vi "MAIN_call.vi"(8 "error IO":errorcluster, 9 "Coordenadas_estacion_input":T1, 10 "Modo":T2=enum."MOVIMIENTO MANUAL", 11 "VISA SESSION":refnum<visa-resource-name>) -> (0 "error out":errorcluster, 2 "Coordenadas_estacion_outpu":T1)   [LabVIEW 2019]
uses:
  Typedefs/Distancia_Z.ctl
  Typedefs/Tipo_movimiento.ctl
  Typedefs/ESTADOS.ctl
  LABVIEW_ROBOT_MASTER/Type_defs/TAREAS_ROBOT.ctl
  LVPROJ_CONFIG_ESTACION/Type_defs/Coordenadas_estacion.ctl
  Typedefs/Distancia.ctl
  Typedefs/Cluster_tracking.ctl
  Typedefs/Cluster_refs_controles.ctl
  SHARED TYPES/Acciones_UI.ctl
  LVPROJ_CONFIG_ESTACION/Type_defs/coordenada_elegida.ctl
  Typedefs/Comandos.ctl
  Typedefs/Estados_arduino.ctl
  <vilib>/Utility/error.llb/Error Cluster From Error Code.vi
  <vilib>/ErrorRing/Error Ring.xnode
  SHARED TYPES/SHARED TYPES.lvlib
  SHARED VI'S/SHARED VI'S.lvlib
panel:
  in  "TabDepuracion":enum32{"Page 1", "Page 2"}(tab)
  out "Config estación?":bool
  in  "Tab Control":enum32{"Page 1"}(tab)
  in  "Set coord. NOK":bool
  in  "Set coord. OK":bool
  in  "Set coord. entrada":bool
  out "Coord.Adquirida Z":u32
  out "Coord.Adquirida Y":u32
  out "Coord.Adquirida X":u32
  in  "Set coord. socket":bool
  out "Tracking_Z":u32
  in  "Distancia Z":T3=32000 items=["2cm"=64000, "1cm"=32000, "1mm"=3200, "0.5mm"=1600, "0.2mm"=640, "0.1mm"=320, "0.05mm"=160]
  out "Movimiento ejecutado?":bool caption="MOVIMIENTO NO EJECUTADO"
  out "Tracking_Y":u32
  out "Tracking_X":u32
  out "TRAMA DE MOVIMIENTO ENVIADA":string
  out "MENSAJES AL USUARIO":string
  in  "COMENZAR MOVIMIENTO":bool
  in  "HOME":bool
  in  "Avance":bool
  in  "Retroceso":bool
  in  "Derecha":bool
  in  "Izquierda":bool
  in  "STOP PROGRAM":bool
  in  "Sube Z":bool
  in  "Baja Z":bool
  out "ESTADO FSM":T4
  out "MOVIMIENTO SOLICITADO":T5=enum."AVANZAR"
  in  "Distancia":T6=9100 items=["60cm"=54600, "50cm"=45500, "45cm"=40950, "40cm"=36400, "35cm"=31850, "30cm"=27300, "25cm"=22750, "20cm"=18200, "15cm"=13650, "10cm"=9100, "5cm"=4550, "2cm"=1820, "1cm"=910, "5mm"=455, "2mm"=182, "1mm"=91, "0.5mm"=45, "0.1mm"=9, "1 paso "=1]
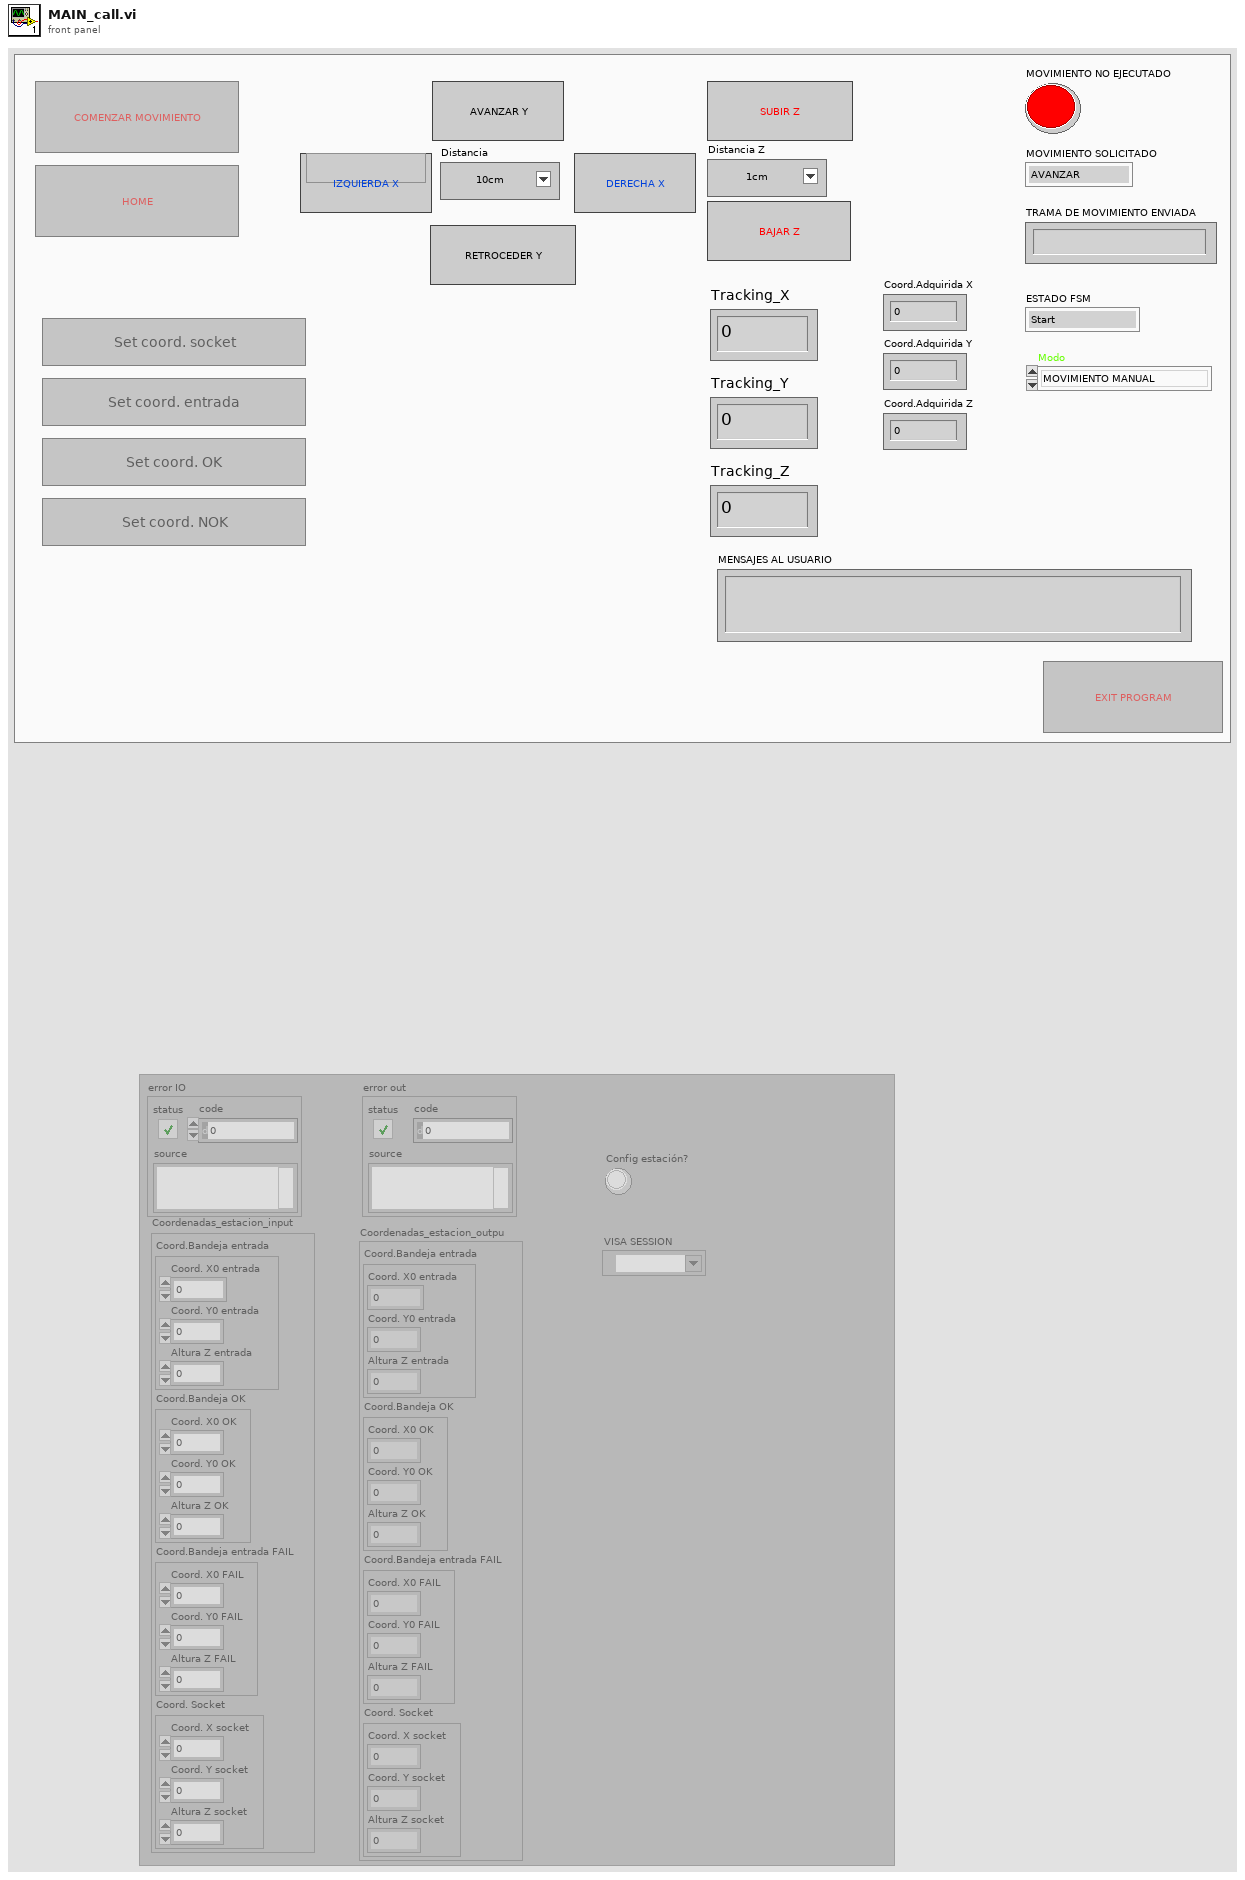
[diagram p1: front panel]
types:
  T1 = typedef "Coordenadas_estacion.ctl" = cluster{"Coord.Bandeja entrada":cluster{"Coord. X0 entrada":u32, "Coord. Y0 entrada ":u32, "Altura Z entrada":u32}, "Coord.Bandeja OK":cluster{"Coord. X0 OK":u32, "Coord. Y0 OK":u32, "Altura Z OK":u32}, "Coord.Bandeja entrada FAIL":cluster{"Coord. X0 FAIL":u32, "Coord. Y0 FAIL":u32, "Altura Z FAIL":u32}, "Coord. Socket":cluster{"Coord. X socket":u32, "Coord. Y socket":u32, "Altura Z socket":u32}}
  T2 = typedef "TAREAS_ROBOT.ctl" = enum16{"NINGUNA", "TEST ASICS", "AJUSTE CAM", "MOVER ASICS", "MOVIMIENTO MANUAL", "LEER QR", "CONFIG ESTACION"}
  T3 = typedef "Distancia_Z.ctl" = i32
  T4 = typedef "ESTADOS.ctl" = enum16{"Start", "Ping_Arduino", "Init Refs", "Check Button", "Check Limits", "Home", "Cabezal Posicion Inicio", "Terminaste posicion inicio?", "Terminar", "Salir Arduino", "Envio Parametros Movimiento", "Recepcion Comando?", "Terminaste Movimiento?", "Adquirir Coordenada", "Terminaste Home?", "Salir"}
  T5 = typedef "Tipo_movimiento.ctl" = enum16{"NINGUNO", "AVANZAR", "RETROCEDER", "DERECHA", "IZQUIERDA", "SUBIRZ", "BAJARZ", "HOME", "HOME_Z"}
  T6 = typedef "Distancia.ctl" = i32
  T7 = typedef "SHARED TYPES.lvlib/Acciones_UI.ctl" = enum16{"Activar", "Desactivar", "Reiniciar default"}
  T8 = typedef "coordenada_elegida.ctl" = enum16{"Ninguna", "Coord.bandeja entrada", "Coord.bandeja OK", "Coord.bandeja FAIL", "Coord.Socket"}
  T9 = enum8{"Enabled", "Disabled", "Disabled and Grayed Out"}
  T10 = typedef "Estados_arduino.ctl" = enum16{"2", "3", "4", "5", "6", "7", "9", "8"}
  T11 = typedef "Comandos.ctl" = enum16{"H", "FH", "FM", "FI", "FX", "FY", "FZ", "I", "OK"}
  T12 = typedef "Cluster_refs_controles.ctl" = cluster{"Comenzar mov":refnum<vi>, "Home":refnum<vi>, "Izq":refnum<vi>, "Der":refnum<vi>, "Stop Program":refnum<vi>, "Avanzar":refnum<vi>, "Bajar Z":refnum<vi>, "Distancia":refnum<vi>, "Subir Z":refnum<vi>, "Retroc":refnum<vi>, "MENSAJES AL USUARIO":refnum<vi>, "Trama enviada":refnum<vi>, "Movimiento ejecutado?":refnum<vi>}
  T13 = typedef "Cluster_tracking.ctl" = cluster{"PasosAcumulados_Y":i32, "PasosAcumulados_X":i32, "PasosAcumulados_Z":i32, "Coord.Adquirida_X":i32, "Coord.Adquirida_Y":i32, "Coord.Adquirida_Z":i32}
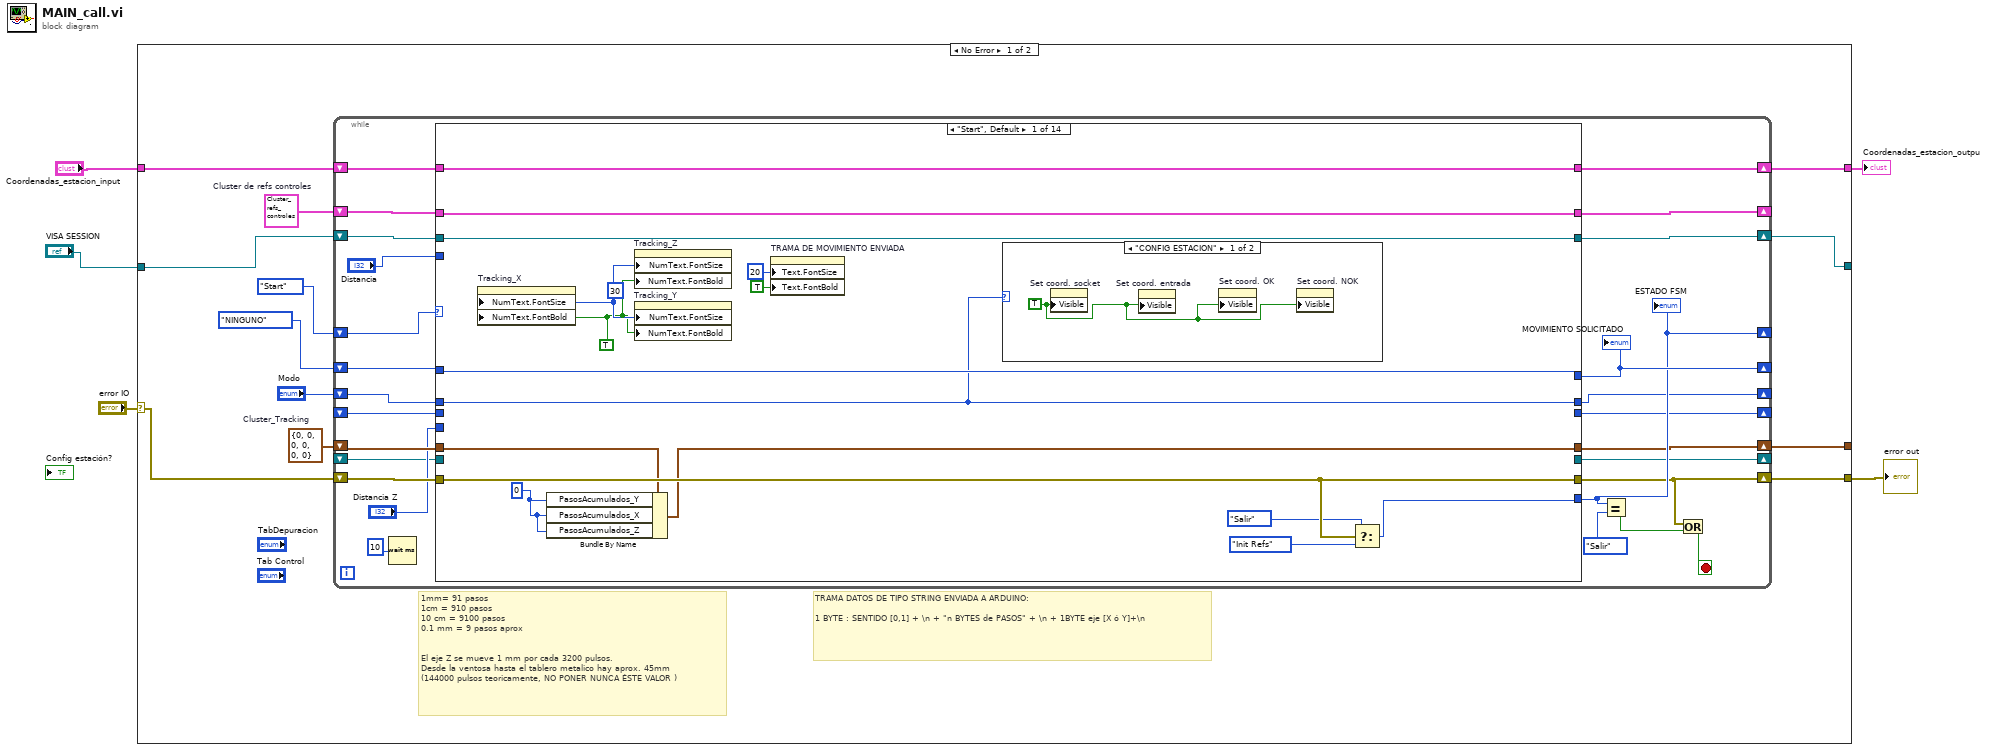
[diagram p0: block diagram]
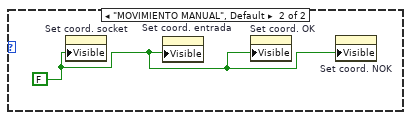
[diagram p2: hidden frame]
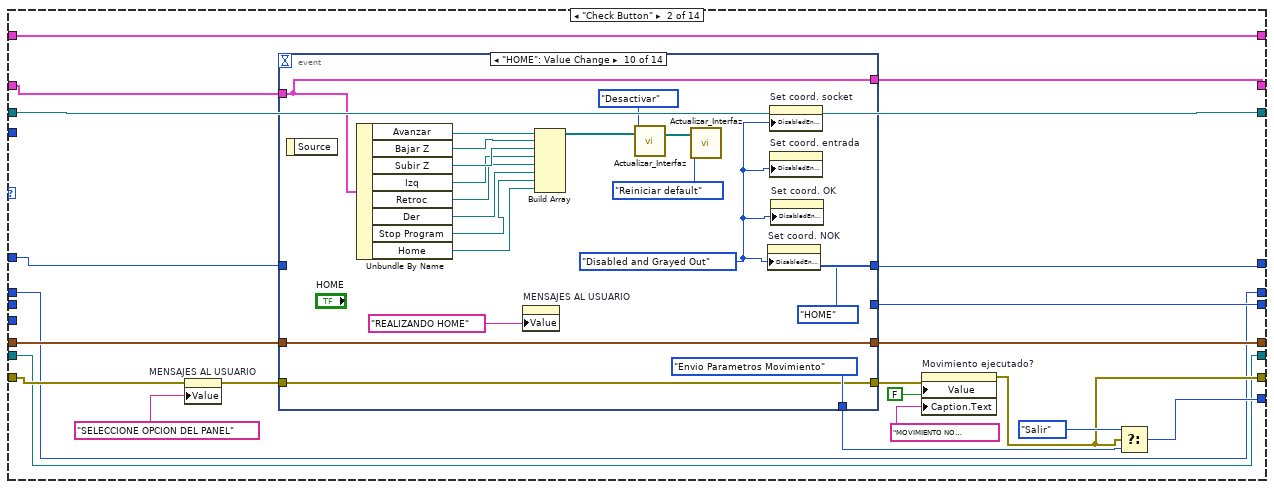
[diagram p3: hidden frame]
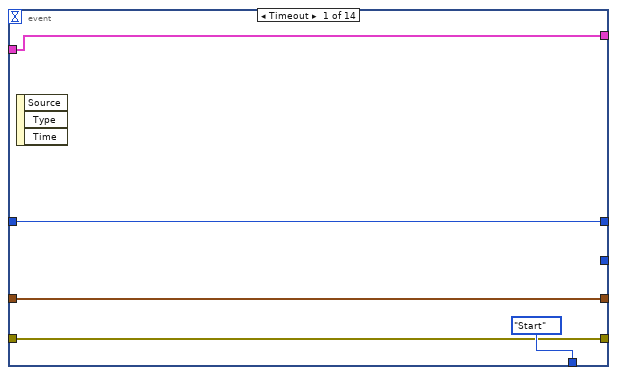
[diagram p4: hidden frame]
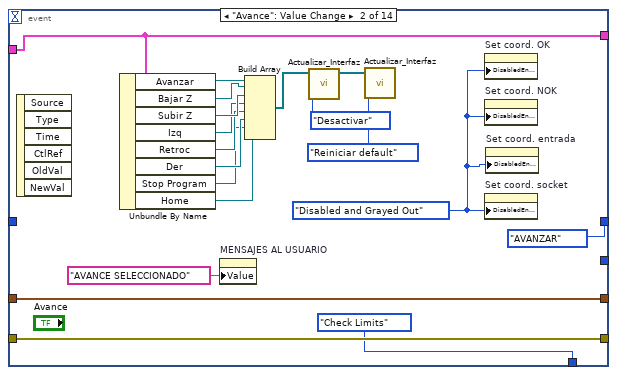
[diagram p5: hidden frame]
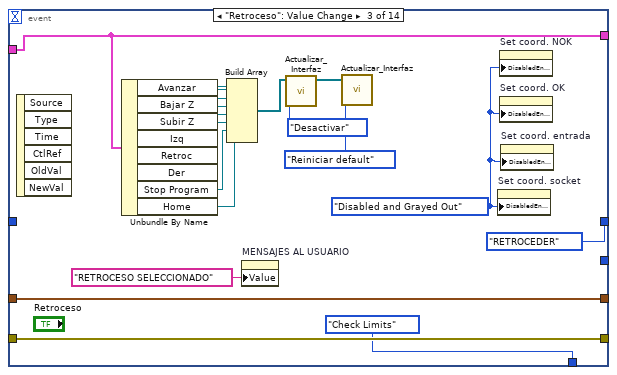
[diagram p6: hidden frame]
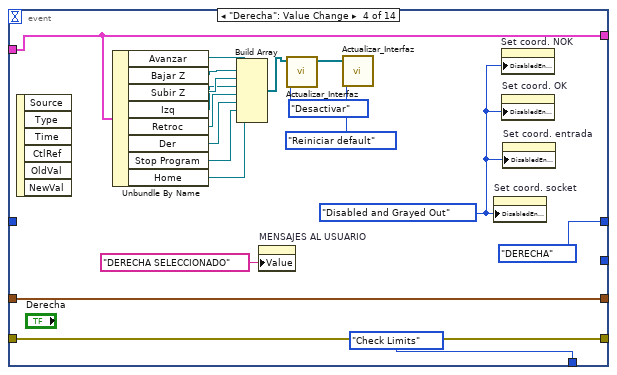
[diagram p7: hidden frame]
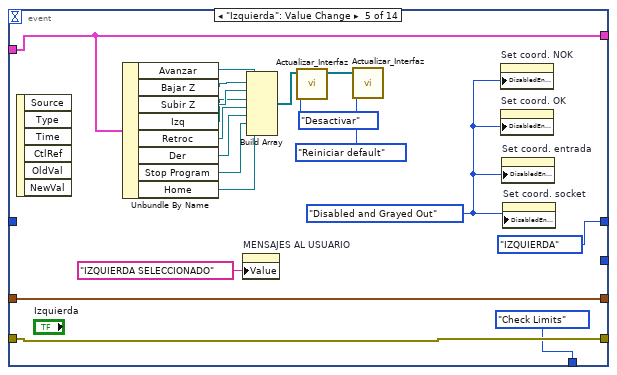
[diagram p8: hidden frame]
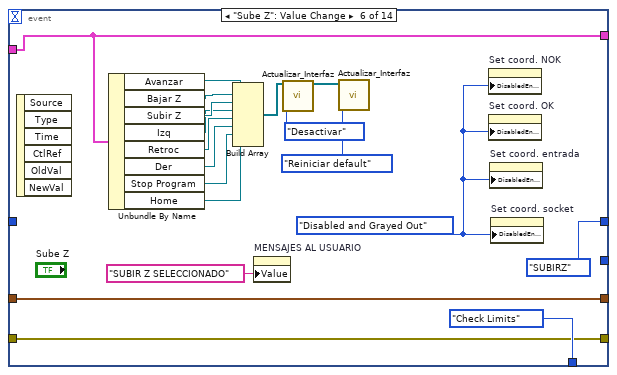
[diagram p9: hidden frame]
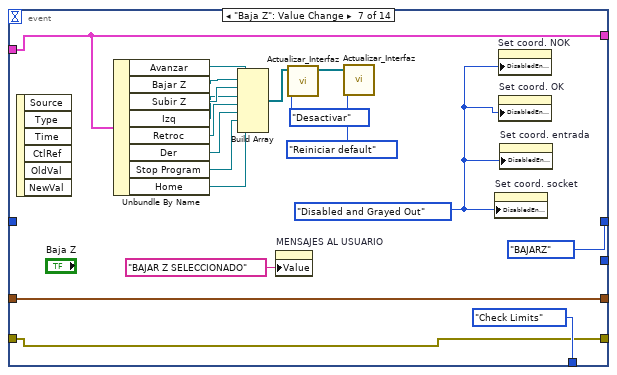
[diagram p10: hidden frame]
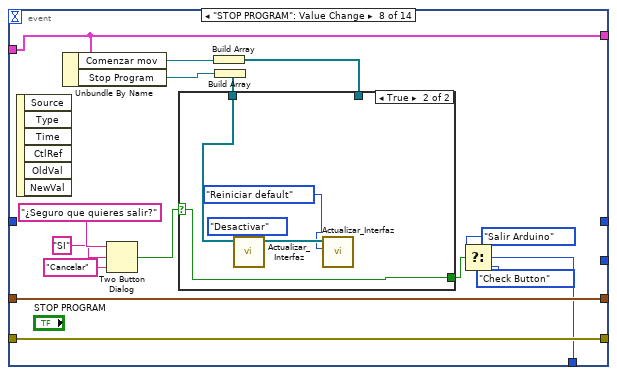
[diagram p11: hidden frame]
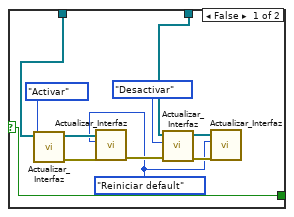
[diagram p12: hidden frame]
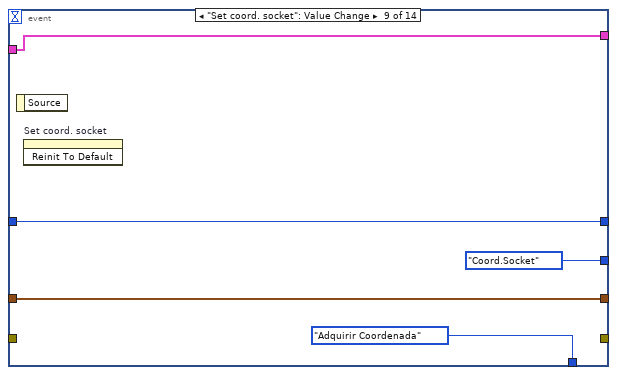
[diagram p13: hidden frame]
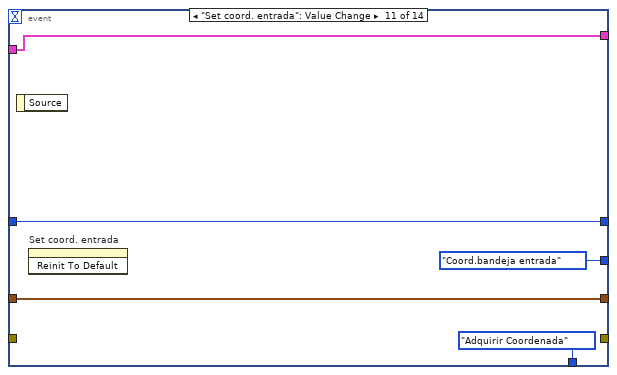
[diagram p14: hidden frame]
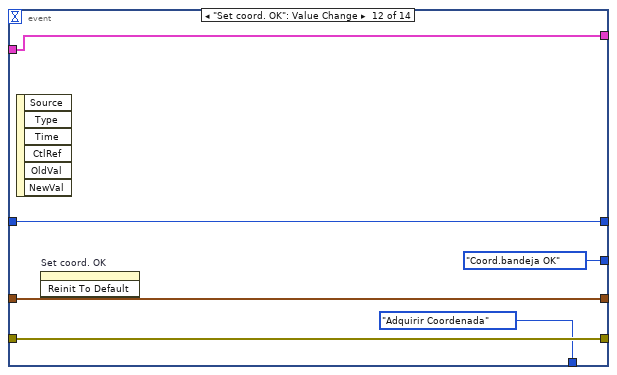
[diagram p15: hidden frame]
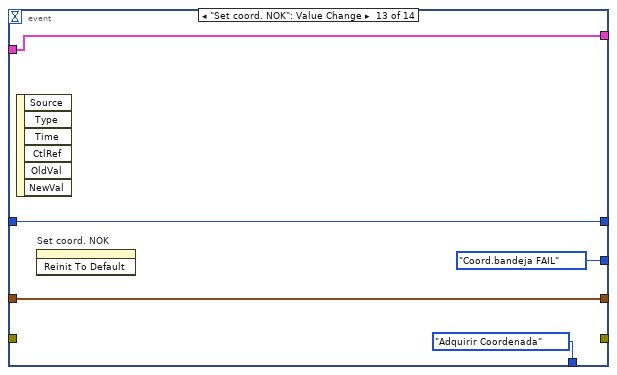
[diagram p16: hidden frame]
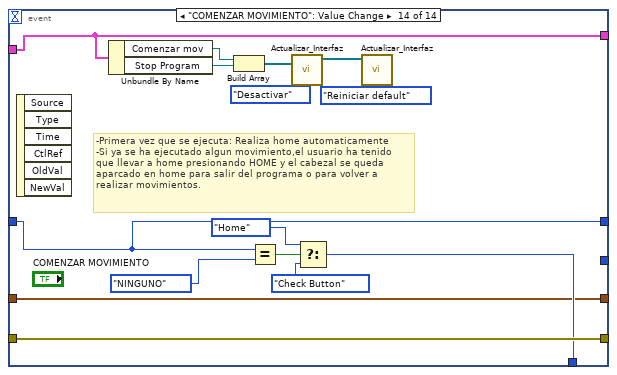
[diagram p17: hidden frame]
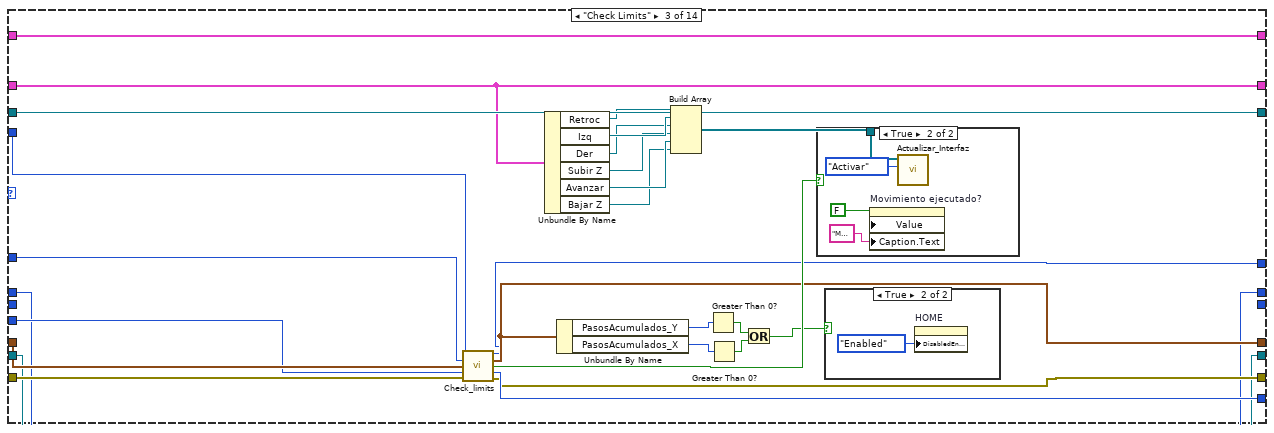
[diagram p18: hidden frame]
diagram:
  n1 = case shown="No Error" "error IO" {
    selector: "error IO" -> [w13 w731]
    tunnel: [w12 w731] -> w4
    tunnel: [w11 _] -> _
    tunnel: "Coordenadas_estacion_input" -> [w9 w730]
    tunnel: [w8 w730] -> w2
    tunnel: "VISA SESSION" -> [w7 w729]
    tunnel: [w6 w729] -> _
    frame No Error {
      w15 = T12 {"Comenzar mov"=refnum, "Home"=refnum, "Izq"=refnum, "Der"=refnum, "Stop Program"=refnum, "Avanzar"=refnum, "Bajar Z"=refnum, "Distancia"=refnum, "Subir Z"=refnum, "Retroc"=refnum, "MENSAJES AL USUARIO"=refnum, "Trama enviada"=refnum, "Movimiento ejecutado?"=refnum}  # Cluster de refs controles
      w14 = T13 {"PasosAcumulados_Y"=0, "PasosAcumulados_X"=0, "PasosAcumulados_Z"=0, "Coord.Adquirida_X"=0, "Coord.Adquirida_Y"=0, "Coord.Adquirida_Z"=0}  # Cluster_Tracking
      # "1mm= 91 pasos\n1cm = 910 pasos\n10 cm = 9100 pasos\n0.1 mm = 9 pasos aprox\n\n\nEl eje Z se mueve 1 mm por cada 3200 pulsos. \nDesde la ventosa hasta el tablero metalico hay aprox. 45mm \n(144000 pulsos teoricamente, NO PONER NUNCA ÉSTE VALOR )"
      # "TRAMA DATOS DE TIPO STRING ENVIADA A ARDUINO:\n\n1 BYTE : SENTIDO [0,1] + \\n + \"n BYTES de PASOS\" + \\n + 1BYTE eje [X ó Y]+\\n"
      n2 = while {
        shift-right: [w31] -> w12
        shift-left: w13 -> [w40]
        shift-right: [w39] -> w6
        shift-left: w7 -> [w41]
        shift-right: [w35] -> _
        shift-left: w15 -> [w36]
        shift-right: [w33] -> _
        shift-left: ESTADOS."Start" ("Enum") -> [w42]
        shift-right: [w37] -> _
        shift-left: Tipo_movimiento."NINGUNO" ("Enum") -> [w38]
        shift-right: [w28] -> w11
        shift-left: w14 -> [w29]
        shift-right: [w24] -> w8
        shift-left: w9 -> [w25]
        shift-right: [w23] -> _
        shift-left: _ -> [w22]
        shift-right: [w20] -> _
        shift-left: "Modo" -> [w26]
        shift-right: [w19] -> _
        shift-left: _ -> [w18]
        stop <- w34 stop-if-true
        n3 = Wait (ms)(milliseconds to wait=u32 10) -> ()  [unwired: 1 out]
        n4 = case shown="\"Start\", Default" w42 {
          tunnel: w41 -> [w55 w67 w314 w324 w364 w406 w449 w488 w517 w573 w593 w613 w658 w707]
          tunnel: w40 -> [w59 w66 w312 w323 w373 w405 w448 w486 w516 w569 w595 w614 w667 w706]
          tunnel: [w59 w68 w293 w331 w341 w392 w432 w486 w513 w569 w591 w612 w655 w710] -> w31
          tunnel: [w56 w79 w311 w335 w370 w402 w445 w483 w536 w570 w594 w616 w661 ESTADOS."Salir" ("f")] -> w33
          tunnel: [w55 w67 w314 w324 w364 w406 w450 w488 w537 w573 w593 w613 w658 w707] -> w39
          tunnel: w38 -> [w54 w76 w310 w336 w375 w409 w451 w487 _ _ _ _ _ w718]
          tunnel: "Distancia" -> [_ _ w313 _ _ w408 _ _ _ _ _ _ _ _]
          tunnel: [w54 w78 w291 w336 w375 w391 w444 w487 _ _ _ _ _ w718] -> w37
          tunnel: w36 -> [w50 w82 w309 w332 w361 w396 w428 w489 w531 w587 w592 w615 w660 w719]
          tunnel: [w50 w81 w309 w332 w361 w396 w428 w489 w531 w574 w592 w615 w660 w719] -> w35
          tunnel: w29 -> [w53 w75 w300 w327 w355 w389 w441 w479 w532 w564 w590 w611 w659 w717]
          tunnel: [w52 w74 w295 w327 w352 w389 w440 w478 w532 w564 w590 w611 w659 w717] -> w28
          tunnel: "Distancia Z" -> [_ _ w292 _ _ w390 _ _ _ _ _ _ _ _]
          tunnel: w26 -> [w44 w62 w288 w320 w338 w386 w410 w470 w511 w556 w588 w609 w653 w699]
          tunnel: w25 -> [w45 w65 w290 w322 w340 w388 w417 w477 w515 w559 w589 w610 w657 w704]
          tunnel: [w45 w65 w290 w322 w340 w388 w417 w473 w515 w559 w589 w610 w657 w704] -> w24
          tunnel: [_ w64 _ _ _ _ _ w472 _ _ _ _ _ _] -> w23
          tunnel: w22 -> [_ _ _ _ _ _ _ w472 _ _ _ _ _ _]
          tunnel: [w44 w62 w288 w320 w338 w386 w410 w470 w511 w556 w588 w609 w653 w699] -> w20
          tunnel: [_ w63 w289 w321 w339 w387 w411 w471 w512 _ _ _ w654 _] -> w19
          tunnel: w18 -> [_ w63 w289 w321 w339 w387 w411 w471 w512 _ _ _ _ w703]
          frame "Start", Default {
            w49 = u32 30 ("Text.Font:Size")
            w48 = TRUE ("Text.Font:Bold")
            w51 = 0 ("PasosAcumulados_Y")
            n5 = property on="Tracking_X" class="DigNum (strict)"("NumText.FontSize"=w49, "NumText.FontBold"=w48) -> ()  [unwired: 2 in, 2 out]
            n6 = Bundle By Name(cluster=w53, "PasosAcumulados_Y"=w51, "PasosAcumulados_X"=w51, "PasosAcumulados_Z"=w51) -> (w52:T13)
            n7 = property on="Tracking_Z" class="DigNum (strict)"("NumText.FontSize"=w49, "NumText.FontBold"=w48) -> ()  [unwired: 2 in, 2 out]
            n8 = property on="Tracking_Y" class="DigNum (strict)"("NumText.FontSize"=w49, "NumText.FontBold"=w48) -> ()  [unwired: 2 in, 2 out]
            n9 = property on="TRAMA DE MOVIMIENTO ENVIADA" class="Str"("Text.FontSize"=u32 20 ("Text.Font:Size"), "Text.FontBold"=TRUE ("Text.Font:Bold")) -> ()  [unwired: 2 in, 2 out]
            n10 = case shown="\"CONFIG ESTACION\"" w44 {
              frame "CONFIG ESTACION" {
                w60 = TRUE ("Visible")
                n11 = property on="Set coord. socket" class="Bool"("Visible"=w60) -> ()  [unwired: 2 in, 2 out]
                n12 = property on="Set coord. entrada" class="Bool"("Visible"=w60) -> ()  [unwired: 2 in, 2 out]
                n13 = property on="Set coord. OK" class="Bool"("Visible"=w60) -> ()  [unwired: 2 in, 2 out]
                n14 = property on="Set coord. NOK" class="Bool"("Visible"=w60) -> ()  [unwired: 2 in, 2 out]
              }
              frame "MOVIMIENTO MANUAL", Default {
                w61 = FALSE ("Visible")
                n15 = property on="Set coord. socket" class="Bool"("Visible"=w61) -> ()  [unwired: 2 in, 2 out]
                n16 = property on="Set coord. entrada" class="Bool"("Visible"=w61) -> ()  [unwired: 2 in, 2 out]
                n17 = property on="Set coord. OK" class="Bool"("Visible"=w61) -> ()  [unwired: 2 in, 2 out]
                n18 = property on="Set coord. NOK" class="Bool"("Visible"=w61) -> ()  [unwired: 2 in, 2 out]
              }
            }
            n19 = Select(t=ESTADOS."Salir", s=w59, f=ESTADOS."Init Refs" ("Enum")) -> (s? t:f=w56:T4)
          }
          frame "Check Button" {
            n20 = property on="MENSAJES AL USUARIO" class="Str"(error in=w66, "Value"="SELECCIONE OPCION DEL PANEL" ("MENSAJES AL USUARIO")) -> (error out=w73:errorcluster)  [unwired: 1 in, 1 out]
            n21 = event shown="[9] \"HOME\": Value Change" {
              selector: _ -> [_ _ _ _ _ _ _ _ _ _ _ _ _ _]
              dyn-events: _ -> [_ _ _ _ _ _ _ _ _ _ _ _ _ _]
              timeout: _ -> [_ _ _ _ _ _ _ _ _ _ _ _ _ _]
              tunnel: w82 -> [w87 w106 w116 w135 w152 w169 w188 w216 w234 w244 w257 w262 w272 w284]
              tunnel: [w87 w106 w116 w135 w152 w169 w188 w216 w234 w244 w257 w262 w272 w284] -> w81
              tunnel: [w86 Tipo_movimiento."AVANZAR" Tipo_movimiento."RETROCEDER" Tipo_movimiento."DERECHA" Tipo_movimiento."IZQUIERDA" Tipo_movimiento."SUBIRZ" Tipo_movimiento."BAJARZ" _ w235 Tipo_movimiento."HOME" w258 w263 w268 w276] -> w78
              tunnel: [ESTADOS."Start" ESTADOS."Check Limits" ("f") ESTADOS."Check Limits" ("f") ESTADOS."Check Limits" ("f") ESTADOS."Check Limits" ("f") ESTADOS."Check Limits" ("Enum") ESTADOS."Check Limits" ("Enum") w208 ESTADOS."Adquirir Coordenada" ("f") ESTADOS."Envio Parametros Movimiento" ESTADOS."Adquirir Coordenada" ("f") ESTADOS."Adquirir Coordenada" ("f") ESTADOS."Adquirir Coordenada" ("f") w275] -> w77
              tunnel: [w84 w92 w110 w129 w148 w180 w199 w214 _ w255 _ w265 _ w281] -> w69
              tunnel: w73 -> [w84 w92 w110 w129 w148 w180 w199 w214 _ w255 _ w265 _ w281]
              tunnel: w76 -> [w86 _ _ _ _ _ _ _ w235 _ w258 w263 w268 w276]
              tunnel: w75 -> [w83 w91 w111 w130 w149 w166 w185 w215 w236 w241 w259 w266 w269 w273]
              tunnel: [w83 w91 w111 w130 w149 w166 w185 w215 w236 w241 w259 w266 w269 w273] -> w74
              tunnel: [_ _ _ _ _ _ _ _ coordenada_elegida."Coord.Socket" ("Enum") _ coordenada_elegida."Coord.bandeja entrada" ("Enum") coordenada_elegida."Coord.bandeja OK" ("Enum") coordenada_elegida."Coord.bandeja FAIL" ("Enum") _] -> w64
              event Timeout {
                n22 = event-data() -> ()  [unwired: 1 in, 3 out]
              }
              event "Avance": Value Change {
                w88 = T9."Disabled and Grayed Out" ("Disabled")
                n23 = event-data() -> ()  [unwired: 1 in, 6 out]
                n24 = Unbundle By Name(w106) -> ("Avanzar"=w105:refnum<vi>, "Bajar Z"=w100:refnum<vi>, "Subir Z"=w99:refnum<vi>, "Izq"=w98:refnum<vi>, "Retroc"=w97:refnum<vi>, "Der"=w96:refnum<vi>, "Stop Program"=w95:refnum<vi>, "Home"=w94:refnum<vi>)
                n25 = property on="MENSAJES AL USUARIO" class="Str"("Value"="AVANCE SELECCIONADO" ("MENSAJES AL USUARIO")) -> ()  [unwired: 2 in, 2 out]
                n26 = Build Array(w105, w100, w99, w98, w97, w96, w95, w94) -> (w104:refnum<vi>[])
                n27 = call "Actualizar_Interfaz.vi"("Enum"=Acciones_UI."Desactivar", "Controls"=w104) -> ("Controls 2"=w102:refnum<vi>[])  [unwired: 8 in, 1 out]
                n28 = call "Actualizar_Interfaz.vi"("Enum"=Acciones_UI."Reiniciar default", "Controls"=w102) -> ()  [unwired: 8 in, 2 out]
                n29 = property on="Set coord. OK" class="Bool"("DisabledEnum"=w88) -> ()  [unwired: 2 in, 2 out]
                n30 = property on="Set coord. NOK" class="Bool"("DisabledEnum"=w88) -> ()  [unwired: 2 in, 2 out]
                n31 = property on="Set coord. socket" class="Bool"("DisabledEnum"=w88) -> ()  [unwired: 2 in, 2 out]
                n32 = property on="Set coord. entrada" class="Bool"("DisabledEnum"=w88) -> ()  [unwired: 2 in, 2 out]
              }
              event "Retroceso": Value Change {
                w107 = T9."Disabled and Grayed Out" ("Disabled")
                n33 = event-data() -> ()  [unwired: 1 in, 6 out]
                n34 = Unbundle By Name(w116) -> ("Avanzar"=w125:refnum<vi>, "Bajar Z"=w121:refnum<vi>, "Subir Z"=w120:refnum<vi>, "Izq"=w119:refnum<vi>, "Retroc"=w118:refnum<vi>, "Der"=w117:refnum<vi>, "Stop Program"=w114:refnum<vi>, "Home"=w113:refnum<vi>)
                n35 = Build Array(w125, w121, w120, w119, w118, w117, w114, w113) -> (w115:refnum<vi>[])
                n36 = property on="MENSAJES AL USUARIO" class="Str"("Value"="RETROCESO SELECCIONADO" ("MENSAJES AL USUARIO")) -> ()  [unwired: 2 in, 2 out]
                n37 = call "Actualizar_Interfaz.vi"("Enum"=Acciones_UI."Desactivar", "Controls"=w115) -> ("Controls 2"=w123:refnum<vi>[])  [unwired: 8 in, 1 out]
                n38 = call "Actualizar_Interfaz.vi"("Enum"=Acciones_UI."Reiniciar default", "Controls"=w123) -> ()  [unwired: 8 in, 2 out]
                n39 = property on="Set coord. socket" class="Bool"("DisabledEnum"=w107) -> ()  [unwired: 2 in, 2 out]
                n40 = property on="Set coord. NOK" class="Bool"("DisabledEnum"=w107) -> ()  [unwired: 2 in, 2 out]
                n41 = property on="Set coord. OK" class="Bool"("DisabledEnum"=w107) -> ()  [unwired: 2 in, 2 out]
                n42 = property on="Set coord. entrada" class="Bool"("DisabledEnum"=w107) -> ()  [unwired: 2 in, 2 out]
              }
              event "Derecha": Value Change {
                w126 = T9."Disabled and Grayed Out" ("Disabled")
                n43 = event-data() -> ()  [unwired: 1 in, 6 out]
                n44 = Unbundle By Name(w135) -> ("Avanzar"=w144:refnum<vi>, "Bajar Z"=w140:refnum<vi>, "Subir Z"=w139:refnum<vi>, "Izq"=w138:refnum<vi>, "Retroc"=w137:refnum<vi>, "Der"=w136:refnum<vi>, "Stop Program"=w134:refnum<vi>, "Home"=w132:refnum<vi>)
                n45 = Build Array(w144, w140, w139, w138, w137, w136, w134, w132) -> (w133:refnum<vi>[])
                n46 = property on="MENSAJES AL USUARIO" class="Str"("Value"="DERECHA SELECCIONADO" ("MENSAJES AL USUARIO")) -> ()  [unwired: 2 in, 2 out]
                n47 = call "Actualizar_Interfaz.vi"("Enum"=Acciones_UI."Desactivar", "Controls"=w133) -> ("Controls 2"=w142:refnum<vi>[])  [unwired: 8 in, 1 out]
                n48 = call "Actualizar_Interfaz.vi"("Enum"=Acciones_UI."Reiniciar default", "Controls"=w142) -> ()  [unwired: 8 in, 2 out]
                n49 = property on="Set coord. socket" class="Bool"("DisabledEnum"=w126) -> ()  [unwired: 2 in, 2 out]
                n50 = property on="Set coord. NOK" class="Bool"("DisabledEnum"=w126) -> ()  [unwired: 2 in, 2 out]
                n51 = property on="Set coord. OK" class="Bool"("DisabledEnum"=w126) -> ()  [unwired: 2 in, 2 out]
                n52 = property on="Set coord. entrada" class="Bool"("DisabledEnum"=w126) -> ()  [unwired: 2 in, 2 out]
              }
              event "Izquierda": Value Change {
                w145 = T9."Disabled and Grayed Out" ("Disabled")
                n53 = event-data() -> ()  [unwired: 1 in, 6 out]
                n54 = Unbundle By Name(w152) -> ("Avanzar"=w163:refnum<vi>, "Bajar Z"=w159:refnum<vi>, "Subir Z"=w158:refnum<vi>, "Izq"=w157:refnum<vi>, "Retroc"=w156:refnum<vi>, "Der"=w155:refnum<vi>, "Stop Program"=w154:refnum<vi>, "Home"=w151:refnum<vi>)
                n55 = property on="MENSAJES AL USUARIO" class="Str"("Value"="IZQUIERDA SELECCIONADO" ("MENSAJES AL USUARIO")) -> ()  [unwired: 2 in, 2 out]
                n56 = Build Array(w163, w159, w158, w157, w156, w155, w154, w151) -> (w153:refnum<vi>[])
                n57 = call "Actualizar_Interfaz.vi"("Enum"=Acciones_UI."Desactivar", "Controls"=w153) -> ("Controls 2"=w161:refnum<vi>[])  [unwired: 8 in, 1 out]
                n58 = call "Actualizar_Interfaz.vi"("Enum"=Acciones_UI."Reiniciar default", "Controls"=w161) -> ()  [unwired: 8 in, 2 out]
                n59 = property on="Set coord. NOK" class="Bool"("DisabledEnum"=w145) -> ()  [unwired: 2 in, 2 out]
                n60 = property on="Set coord. OK" class="Bool"("DisabledEnum"=w145) -> ()  [unwired: 2 in, 2 out]
                n61 = property on="Set coord. entrada" class="Bool"("DisabledEnum"=w145) -> ()  [unwired: 2 in, 2 out]
                n62 = property on="Set coord. socket" class="Bool"("DisabledEnum"=w145) -> ()  [unwired: 2 in, 2 out]
              }
              event "Sube Z": Value Change {
                w164 = T9."Disabled and Grayed Out" ("Disabled")
                n63 = event-data() -> ()  [unwired: 1 in, 6 out]
                n64 = Unbundle By Name(w169) -> ("Avanzar"=w179:refnum<vi>, "Bajar Z"=w175:refnum<vi>, "Subir Z"=w174:refnum<vi>, "Izq"=w173:refnum<vi>, "Retroc"=w172:refnum<vi>, "Der"=w171:refnum<vi>, "Stop Program"=w170:refnum<vi>, "Home"=w167:refnum<vi>)
                n65 = Build Array(w179, w175, w174, w173, w172, w171, w170, w167) -> (w168:refnum<vi>[])
                n66 = property on="MENSAJES AL USUARIO" class="Str"("Value"="SUBIR Z SELECCIONADO" ("MENSAJES AL USUARIO")) -> ()  [unwired: 2 in, 2 out]
                n67 = call "Actualizar_Interfaz.vi"("Enum"=Acciones_UI."Desactivar", "Controls"=w168) -> ("Controls 2"=w177:refnum<vi>[])  [unwired: 8 in, 1 out]
                n68 = call "Actualizar_Interfaz.vi"("Enum"=Acciones_UI."Reiniciar default", "Controls"=w177) -> ()  [unwired: 8 in, 2 out]
                n69 = property on="Set coord. NOK" class="Bool"("DisabledEnum"=w164) -> ()  [unwired: 2 in, 2 out]
                n70 = property on="Set coord. OK" class="Bool"("DisabledEnum"=w164) -> ()  [unwired: 2 in, 2 out]
                n71 = property on="Set coord. entrada" class="Bool"("DisabledEnum"=w164) -> ()  [unwired: 2 in, 2 out]
                n72 = property on="Set coord. socket" class="Bool"("DisabledEnum"=w164) -> ()  [unwired: 2 in, 2 out]
              }
              event "Baja Z": Value Change {
                w183 = T9."Disabled and Grayed Out" ("Disabled")
                n73 = event-data() -> ()  [unwired: 1 in, 6 out]
                n74 = Unbundle By Name(w188) -> ("Avanzar"=w198:refnum<vi>, "Bajar Z"=w194:refnum<vi>, "Subir Z"=w193:refnum<vi>, "Izq"=w192:refnum<vi>, "Retroc"=w191:refnum<vi>, "Der"=w190:refnum<vi>, "Stop Program"=w189:refnum<vi>, "Home"=w186:refnum<vi>)
                n75 = Build Array(w198, w194, w193, w192, w191, w190, w189, w186) -> (w187:refnum<vi>[])
                n76 = property on="MENSAJES AL USUARIO" class="Str"("Value"="BAJAR Z SELECCIONADO" ("MENSAJES AL USUARIO")) -> ()  [unwired: 2 in, 2 out]
                n77 = call "Actualizar_Interfaz.vi"("Enum"=Acciones_UI."Desactivar", "Controls"=w187) -> ("Controls 2"=w196:refnum<vi>[])  [unwired: 8 in, 1 out]
                n78 = call "Actualizar_Interfaz.vi"("Enum"=Acciones_UI."Reiniciar default", "Controls"=w196) -> ()  [unwired: 8 in, 2 out]
                n79 = property on="Set coord. socket" class="Bool"("DisabledEnum"=w183) -> ()  [unwired: 2 in, 2 out]
                n80 = property on="Set coord. NOK" class="Bool"("DisabledEnum"=w183) -> ()  [unwired: 2 in, 2 out]
                n81 = property on="Set coord. OK" class="Bool"("DisabledEnum"=w183) -> ()  [unwired: 2 in, 2 out]
                n82 = property on="Set coord. entrada" class="Bool"("DisabledEnum"=w183) -> ()  [unwired: 2 in, 2 out]
              }
              event "STOP PROGRAM": Value Change {
                n83 = event-data() -> ()  [unwired: 1 in, 6 out]
                n84 = Unbundle By Name(w216) -> ("Comenzar mov"=w203:refnum<vi>, "Stop Program"=w207:refnum<vi>)
                n85 = Two Button Dialog(message="¿Seguro que quieres salir?", 1:"Cancelar" ("F button name (\"Cancel\")"), 2:"SI" ("T button name (\"OK\")")) -> (T button?=w206:bool)
                n86 = Build Array(w203) -> (w202:refnum<vi>[])
                n87 = Build Array(w207) -> (w204:refnum<vi>[])
                n88 = case shown="True" w206 {
                  selector: w206 -> [w226 w228]
                  tunnel: w204 -> [w225 w231]
                  tunnel: [w226 w228] -> w205
                  tunnel: w202 -> [w222 _]
                  frame False {
                    w217 = Acciones_UI."Reiniciar default" ("Enum")
                    n89 = call "Actualizar_Interfaz.vi"("Enum"=Acciones_UI."Activar", "Controls"=w225) -> ("error out"=w223:errorcluster, "Controls 2"=w224:refnum<vi>[])  [unwired: 8 in]
                    n90 = call "Actualizar_Interfaz.vi"("error in (no error)"=w223, "Enum"=w217, "Controls"=w224) -> ("error out"=w220:errorcluster)  [unwired: 7 in, 1 out]
                    n91 = call "Actualizar_Interfaz.vi"("error in (no error)"=w220, "Enum"=Acciones_UI."Desactivar", "Controls"=w222) -> ("error out"=w219:errorcluster, "Controls 2"=w221:refnum<vi>[])  [unwired: 7 in]
                    n92 = call "Actualizar_Interfaz.vi"("error in (no error)"=w219, "Enum"=w217, "Controls"=w221) -> ()  [unwired: 7 in, 2 out]
                  }
                  frame True {
                    n93 = call "Actualizar_Interfaz.vi"("Enum"=Acciones_UI."Desactivar", "Controls"=w231) -> ("Controls 2"=w230:refnum<vi>[])  [unwired: 8 in, 1 out]
                    n94 = call "Actualizar_Interfaz.vi"("Enum"=Acciones_UI."Reiniciar default", "Controls"=w230) -> ()  [unwired: 8 in, 2 out]
                  }
                }
                n95 = Select(t=ESTADOS."Salir Arduino" ("Enum"), s=w205, f=ESTADOS."Check Button") -> (s? t:f=w208:T4)
              }
              event "Set coord. socket": Value Change {
                n96 = event-data() -> ()  [unwired: 1 in, 1 out]
                n97 = invoke on="Set coord. socket" class="Bool" method="Reinit To Default"() -> ()  [unwired: 3 in, 3 out]
              }
              event "HOME": Value Change {
                w238 = T9."Disabled and Grayed Out" ("Disabled")
                n98 = event-data() -> ()  [unwired: 1 in, 1 out]
                n99 = Unbundle By Name(w244) -> ("Avanzar"=w253:refnum<vi>, "Bajar Z"=w248:refnum<vi>, "Subir Z"=w247:refnum<vi>, "Izq"=w246:refnum<vi>, "Retroc"=w245:refnum<vi>, "Der"=w239:refnum<vi>, "Stop Program"=w243:refnum<vi>, "Home"=w242:refnum<vi>)
                n100 = property on="MENSAJES AL USUARIO" class="Str"("Value"="REALIZANDO HOME" ("MENSAJES AL USUARIO")) -> ()  [unwired: 2 in, 2 out]
                n101 = Build Array(w253, w248, w247, w246, w245, w239, w243, w242) -> (w252:refnum<vi>[])
                n102 = call "Actualizar_Interfaz.vi"("Enum"=Acciones_UI."Desactivar", "Controls"=w252) -> ("Controls 2"=w250:refnum<vi>[])  [unwired: 8 in, 1 out]
                n103 = call "Actualizar_Interfaz.vi"("Enum"=Acciones_UI."Reiniciar default", "Controls"=w250) -> ()  [unwired: 8 in, 2 out]
                n104 = property on="Set coord. NOK" class="Bool"("DisabledEnum"=w238) -> ()  [unwired: 2 in, 2 out]
                n105 = property on="Set coord. socket" class="Bool"("DisabledEnum"=w238) -> ()  [unwired: 2 in, 2 out]
                n106 = property on="Set coord. entrada" class="Bool"("DisabledEnum"=w238) -> ()  [unwired: 2 in, 2 out]
                n107 = property on="Set coord. OK" class="Bool"("DisabledEnum"=w238) -> ()  [unwired: 2 in, 2 out]
              }
              event "Set coord. entrada": Value Change {
                n108 = event-data() -> ()  [unwired: 1 in, 1 out]
                n109 = invoke on="Set coord. entrada" class="Bool" method="Reinit To Default"() -> ()  [unwired: 3 in, 3 out]
              }
              event "Set coord. OK": Value Change {
                n110 = event-data() -> ()  [unwired: 1 in, 6 out]
                n111 = invoke on="Set coord. OK" class="Bool" method="Reinit To Default"() -> ()  [unwired: 3 in, 3 out]
              }
              event "Set coord. NOK": Value Change {
                n112 = event-data() -> ()  [unwired: 1 in, 6 out]
                n113 = invoke on="Set coord. NOK" class="Bool" method="Reinit To Default"() -> ()  [unwired: 3 in, 3 out]
              }
              event "COMENZAR MOVIMIENTO": Value Change {
                # "-Primera vez que se ejecuta: Realiza home automaticamente\n-Si ya se ha ejecutado algun movimiento,el usuario ha tenido que llevar a home presionando HOME y el cabezal se queda aparcado en home para salir del programa o para volver a realizar movimientos."
                n114 = event-data() -> ()  [unwired: 1 in, 6 out]
                n115 = Unbundle By Name(w284) -> ("Comenzar mov"=w287:refnum<vi>, "Stop Program"=w274:refnum<vi>)
                n116 = Build Array(w287, w274) -> (w286:refnum<vi>[])
                n117 = Equal?(x=w276, y=Tipo_movimiento."NINGUNO") -> (x = y?=w279:bool)
                n118 = call "Actualizar_Interfaz.vi"("Enum"=Acciones_UI."Desactivar", "Controls"=w286) -> ("Controls 2"=w283:refnum<vi>[])  [unwired: 8 in, 1 out]
                n119 = Select(t=ESTADOS."Home", s=w279, f=ESTADOS."Check Button") -> (s? t:f=w275:T4)
                n120 = call "Actualizar_Interfaz.vi"("Enum"=Acciones_UI."Reiniciar default", "Controls"=w283) -> ()  [unwired: 8 in, 2 out]
              }
            }
            n121 = property on="Movimiento ejecutado?" class="Bool (strict)"(error in=w69, "Value"=FALSE ("Movimiento ejecutado?"), "Caption.Text"="MOVIMIENTO NO EJECUTADO" ("Label.Text")) -> (error out=w68:errorcluster)  [unwired: 1 in, 1 out]
            n122 = Select(t=ESTADOS."Salir", s=w68, f=w77) -> (s? t:f=w79:T4)
          }
          frame "Check Limits" {
            n123 = call "Check_limits.vi"("Distancia X/Y"=w313, "Tipo Movimiento"=w310, "Cluster_Tracking"=w300, "Distancia Z"=w292, "error in (no error)"=w312) -> ("Tipo Movimiento 2"=w291:T5, "Cluster_Tracking 2"=w295:T13, "Limite sobrepasado?"=w308:bool, "Estado"=w311:T4, "error out"=w293:errorcluster)  [unwired: 6 in]
            n124 = Unbundle By Name(w309) -> ("Retroc"=w307:refnum<vi>, "Izq"=w306:refnum<vi>, "Der"=w305:refnum<vi>, "Subir Z"=w304:refnum<vi>, "Avanzar"=w303:refnum<vi>, "Bajar Z"=w302:refnum<vi>)
            n125 = Unbundle By Name(w295) -> ("PasosAcumulados_Y"=w298:i32, "PasosAcumulados_X"=w297:i32)
            n126 = Build Array(w307, w306, w305, w304, w303, w302) -> (w301:refnum<vi>[])
            n127 = Greater Than 0?(x=w298) -> (x > 0?=w299:bool)
            n128 = Greater Than 0?(x=w297) -> (x > 0?=w296:bool)
            n129 = Or(x=w299, y=w296) -> (x .or. y?=w294:bool)
            n130 = case shown="True" w308 {
              tunnel: w301 -> [_ w319]
              frame False {
              }
              frame True {
                n131 = property on="Movimiento ejecutado?" class="Bool (strict)"("Value"=FALSE ("Movimiento ejecutado"), "Caption.Text"="MOVIMIENTO NO EJECUTADO" ("Label.Text")) -> ()  [unwired: 2 in, 2 out]
                n132 = call "Actualizar_Interfaz.vi"("Enum"=Acciones_UI."Activar", "Controls"=w319) -> ()  [unwired: 8 in, 2 out]
              }
            }
            n133 = case shown="True" w294 {
              frame False {
              }
              frame True {
                n134 = property on="HOME" class="Bool"("DisabledEnum"=T9."Enabled" ("Disabled")) -> ()  [unwired: 2 in, 2 out]
              }
            }
          }
          frame "Home" {
            # "LEO ESTADO EN ARDUINO"
            # "ROBOT SE MUEVE:\nHACE HOME"
            n135 = call "Ack_estado_Arduino.vi"("error in (no error)"=w323, "Enum"=Estados_arduino."2", "VISA resource name"=w324) -> ("error out"=w337:errorcluster)  [unwired: 6 in, 2 out]
            n136 = call "Enviar_comando.vi"("error in (no error)"=w337, "Enum"=Comandos."H", "VISA resource name"=w324) -> ("error out"=w330:errorcluster)  [unwired: 6 in, 2 out]
            n137 = Unbundle By Name(w332) -> ("MENSAJES AL USUARIO"=w329:refnum<vi>)
            n138 = property class="Str"(reference=w329, error in=w330, "Text.Text"="HACIENDO HOME") -> (error out=w331:errorcluster)  [unwired: 1 out]
            n139 = Select(t=ESTADOS."Start" ("Enum"), s=w331, f=ESTADOS."Terminaste Home?" ("Enum")) -> (s? t:f=w335:T4)
          }
          frame "Terminar" {
            w344 = 0 ("PasosAcumulados_Y")
            # "LEO ESTADO EN ARDUINO"
            # "ESPERAR A QUE HAGA HOME Y NOS ENVIE EL COMANDO\nDE FINISHED HOME"
            n140 = call "Ack_estado_Arduino.vi"("error in (no error)"=w373, "Enum"=Estados_arduino."2", "VISA resource name"=w364) -> ("error out"=w369:errorcluster)  [unwired: 6 in, 2 out]
            n141 = Bundle By Name(cluster=w355, "PasosAcumulados_Y"=w344, "PasosAcumulados_X"=w344, "PasosAcumulados_Z"=w344) -> (w352:T13)
            n142 = call "Enviar_comando.vi"("error in (no error)"=w369, "Enum"=Comandos."H", "VISA resource name"=w364) -> ("error out"=w363:errorcluster)  [unwired: 6 in, 2 out]
            n143 = call "Ack_estado_Arduino.vi"("error in (no error)"=w363, "Enum"=Estados_arduino."3", "VISA resource name"=w364) -> ("error out"=w365:errorcluster)  [unwired: 6 in, 2 out]
            n144 = case shown="No Error" w365 {
              selector: w365 -> [w376 w385]
              tunnel: [w378 w385] -> w367
              tunnel: w364 -> [w377 _]
              frame No Error {
                n145 = while {
                  tunnel: [w384] -> w378
                  tunnel: w377 -> [w380]
                  tunnel: w376 -> [w379]
                  stop <- w381 stop-if-true
                  n146 = property class="Instr"(reference=w380, error in=w379) -> (error out=w384:errorcluster, "Serial Settings:Number of Bytes at Serial Port"=w383:u32)  [unwired: 1 out]
                  n147 = Equal?(x=w383, y=u32 2) -> (x = y?=w381:bool)
                }
              }
              frame Error {
              }
            }
            n148 = Unbundle By Name(w361) -> ("Izq"=w360:refnum<vi>, "Stop Program"=w356:refnum<vi>, "Avanzar"=w349:refnum<vi>, "Bajar Z"=w348:refnum<vi>, "Der"=w347:refnum<vi>, "Subir Z"=w346:refnum<vi>, "Retroc"=w345:refnum<vi>)
            n149 = call "Ack_comando_arduino.vi"("error in (no error)"=w367, 10:Comandos."FH", "VISA resource name"=w364) -> ("error IO"=w359:errorcluster)  [unwired: 6 in, 2 out]
            n150 = Unbundle By Name(w352) -> ("PasosAcumulados_X"=w351:i32, "PasosAcumulados_Y"=w350:i32, "PasosAcumulados_Z"=w342:i32)
            n151 = Build Array(w360, w356, w349, w348, w347, w346, w345) -> (w358:refnum<vi>[])
            n152 = call "Actualizar_Interfaz.vi"("error in (no error)"=w359, "Enum"=Acciones_UI."Activar", "Controls"=w358) -> ("error out"=w354:errorcluster)  [unwired: 7 in, 1 out]
            n153 = property on="Tracking_X" class="DigNum (strict)"(error in=w354, "Value"=w351) -> (error out=w353:errorcluster)  [unwired: 1 in, 1 out]
            n154 = property on="Tracking_Y" class="DigNum (strict)"(error in=w353, "Value"=w350) -> (error out=w343:errorcluster)  [unwired: 1 in, 1 out]
            n155 = property on="Tracking_Z" class="DigNum (strict)"(error in=w343, "Value"=w342) -> (error out=w341:errorcluster)  [unwired: 1 in, 1 out]
            n156 = Select(t=ESTADOS."Salir" ("Enum"), s=w341, f=ESTADOS."Check Button") -> (s? t:f=w370:T4)
          }
          frame "Envio Parametros Movimiento" {
            n157 = call "Ack_estado_Arduino.vi"("error in (no error)"=w405, "Enum"=Estados_arduino."6", "VISA resource name"=w406) -> ("error out"=w404:errorcluster)  [unwired: 6 in, 2 out]
            n158 = call "Enviar_trama_movimiento.vi"("VISA resource name"=w406, "Cluster_Tracking"=w389, "Tipo movimiento"=w409, "Distancia Z"=w390, "Distancia X/Y"=w408, "error in (no error)"=w404) -> ("TRAMA ENVIADA"=w394:string, "Tipo movimiento"=w391:T5, "error out"=w395:errorcluster)  [unwired: 6 in, 1 out]
            n159 = Unbundle By Name(w396) -> ("Trama enviada"=w393:refnum<vi>)
            n160 = Equal?(x=w391, y=Tipo_movimiento."HOME") -> (x = y?=w400:bool)
            n161 = property class="Str"(reference=w393, error in=w395, "Text.Text"=w394) -> (error out=w392:errorcluster)  [unwired: 1 out]
            n162 = Select(t=ESTADOS."Terminar", s=w400, f=ESTADOS."Terminaste Movimiento?") -> (s? t:f=w397:T4)
            n163 = Select(t=ESTADOS."Salir" ("Enum"), s=w392, f=w397) -> (s? t:f=w402:T4)
          }
          frame "Terminaste Movimiento?" {
            w412 = T9."Enabled" ("Disabled")
            n164 = call "check_finalMovimiento.vi"("error in (no error)"=w448, "Cluster_Tracking in"=w441, "Enum in"=w451, "VISA Refnum in"=w449) -> ("error out"=w419:errorcluster, "Cluster_Tracking out"=w440:T13, "Enum out"=w444:T5, "VISA Refnum out"=w450:refnum<visa-resource-name>, "Movimiento realizado?"=w429:bool)  [unwired: 3 in]
            n165 = property on="Set coord. socket" class="Bool"(error in=w419, "DisabledEnum"=w412) -> (error out=w416:errorcluster)  [unwired: 1 in, 1 out]
            n166 = property on="Movimiento ejecutado?" class="Bool (strict)"("Value"=w429, "Caption.Text"="MOVIMIENTO EJECUTADO" ("Label.Text")) -> ()  [unwired: 2 in, 2 out]
            n167 = property on="Set coord. NOK" class="Bool"(error in=w416, "DisabledEnum"=w412) -> (error out=w415:errorcluster)  [unwired: 1 in, 1 out]
            n168 = Unbundle By Name(w440) -> ("PasosAcumulados_X"=w439:i32, "PasosAcumulados_Y"=w438:i32, "PasosAcumulados_Z"=w433:i32)
            n169 = property on="Set coord. OK" class="Bool"(error in=w415, "DisabledEnum"=w412) -> (error out=w414:errorcluster)  [unwired: 1 in, 1 out]
            n170 = Unbundle By Name(w428) -> ("Der"=w427:refnum<vi>, "Izq"=w426:refnum<vi>, "Avanzar"=w425:refnum<vi>, "Retroc"=w424:refnum<vi>, "Subir Z"=w423:refnum<vi>, "Bajar Z"=w422:refnum<vi>)
            n171 = property on="Set coord. entrada" class="Bool"(error in=w414, "DisabledEnum"=w412) -> (error out=w413:errorcluster)  [unwired: 1 in, 1 out]
            n172 = Build Array(w427, w426, w425, w424, w423, w422) -> (w421:refnum<vi>[])
            n173 = Not Equal To 0?(x=w439) -> (x != 0?=w437:bool)
            n174 = Not Equal To 0?(x=w438) -> (x != 0?=w436:bool)
            n175 = Not Equal To 0?(x=w433) -> (x != 0?=w435:bool)
            n176 = call "Actualizar_Interfaz.vi"("error in (no error)"=w413, "Enum"=Acciones_UI."Activar", "Controls"=w421) -> ("error out"=w418:errorcluster)  [unwired: 7 in, 1 out]
            n177 = Compound Arithmetic op=OR(w437, w436, w435) -> (w434:bool)
            n178 = case shown="True" w434 {
              tunnel: w418 -> [w456 w466]
              tunnel: [w454 w466] -> w431
              tunnel: w428 -> [w453 w465]
              frame False {
                n179 = Unbundle By Name(w453) -> ("Stop Program"=w457:refnum<vi>, "Home"=w461:refnum<vi>)
                n180 = Build Array(w461) -> (w460:refnum<vi>[])
                n181 = call "Actualizar_Interfaz.vi"("error in (no error)"=w456, "Enum"=Acciones_UI."Desactivar", "Controls"=w460) -> ("error out"=w455:errorcluster)  [unwired: 7 in, 1 out]
                n182 = Build Array(w457) -> (w452:refnum<vi>[])
                n183 = call "Actualizar_Interfaz.vi"("error in (no error)"=w455, "Enum"=Acciones_UI."Activar", "Controls"=w452) -> ("error out"=w454:errorcluster)  [unwired: 7 in, 1 out]
              }
              frame True {
                n184 = Unbundle By Name(w465) -> ("Stop Program"=w464:refnum<vi>, "Home"=w469:refnum<vi>)
                n185 = Build Array(w469) -> (w467:refnum<vi>[])
                n186 = call "Actualizar_Interfaz.vi"("Enum"=Acciones_UI."Activar", "Controls"=w467) -> ()  [unwired: 8 in, 2 out]
                n187 = Build Array(w464) -> (w462:refnum<vi>[])
                n188 = call "Actualizar_Interfaz.vi"("Enum"=Acciones_UI."Desactivar", "Controls"=w462) -> ()  [unwired: 8 in, 2 out]
              }
            }
            n189 = property on="Tracking_X" class="DigNum (strict)"(error in=w431, "Value"=w439) -> (error out=w443:errorcluster)  [unwired: 1 in, 1 out]
            n190 = property on="Tracking_Y" class="DigNum (strict)"(error in=w443, "Value"=w438) -> (error out=w442:errorcluster)  [unwired: 1 in, 1 out]
            n191 = property on="Tracking_Z" class="DigNum (strict)"(error in=w442, "Value"=w433) -> (error out=w432:errorcluster)  [unwired: 1 in, 1 out]
            n192 = Select(t=ESTADOS."Salir" ("Enum"), s=w432, f=ESTADOS."Check Button") -> (s? t:f=w445:T4)
          }
          frame "Adquirir Coordenada" {
            n193 = Unbundle By Name(w479) -> ("PasosAcumulados_Y"=w482:i32, "PasosAcumulados_X"=w481:i32, "PasosAcumulados_Z"=w480:i32)
            n194 = Bundle By Name(cluster=w479, "Coord.Adquirida_Y"=w482, "Coord.Adquirida_X"=w481, "Coord.Adquirida_Z"=w480) -> (w478:T13)
            n195 = Unbundle By Name(w478) -> ("Coord.Adquirida_X"=w476:i32, "Coord.Adquirida_Y"=w475:i32, "Coord.Adquirida_Z"=w474:i32)
            "Coord.Adquirida X" <- w476
            "Coord.Adquirida Y" <- w475
            "Coord.Adquirida Z" <- w474
            n196 = case shown="\"Coord.bandeja FAIL\"" w472 {
              tunnel: w477 -> [w490 w495 w500 w505 w510]
              tunnel: [w490 w494 w499 w504 w509] -> w473
              tunnel: w476 -> [_ w493 w498 w503 w508]
              tunnel: w475 -> [_ w492 w497 w502 w507]
              tunnel: w474 -> [_ w491 w496 w501 w506]
              frame "Ninguna", Default {
              }
              frame "Coord.bandeja entrada" {
                n197 = Bundle By Name(cluster=w495, "Coord.Bandeja entrada.Coord. X0 entrada"=w493, "Coord.Bandeja entrada.Coord. Y0 entrada"=w492, "Coord.Bandeja entrada.Altura Z entrada"=w491) -> (w494:T1)
              }
              frame "Coord.bandeja OK" {
                n198 = Bundle By Name(cluster=w500, "Coord.Bandeja OK.Coord. X0 OK"=w498, "Coord.Bandeja OK.Coord. Y0 OK"=w497, "Coord.Bandeja OK.Altura Z OK"=w496) -> (w499:T1)
              }
              frame "Coord.bandeja FAIL" {
                n199 = Bundle By Name(cluster=w505, "Coord.Bandeja entrada FAIL.Coord. X0 FAIL"=w503, "Coord.Bandeja entrada FAIL.Coord. Y0 FAIL"=w502, "Coord.Bandeja entrada FAIL.Altura Z FAIL"=w501) -> (w504:T1)
              }
              frame "Coord.Socket" {
                n200 = Bundle By Name(cluster=w510, "Coord. Socket.Coord. X socket"=w508, "Coord. Socket.Coord. Y socket"=w507, "Coord. Socket.Altura Z socket"=w506) -> (w509:T1)
              }
            }
            n201 = Select(t=ESTADOS."Salir", s=w486, f=ESTADOS."Check Button" ("y")) -> (s? t:f=w483:T4)
          }
          frame "Terminaste Home?" {
            w514 = T9."Enabled" ("Disabled")
            # "LEO ESTADO EN ARDUINO"
            # "ESPERAR A QUE HAGA HOME Y NOS ENVIE EL COMANDO\nDE FINISHED HOME \"FH\""
            n202 = call "Ack_estado_Arduino.vi"("error in (no error)"=w516, "Enum"=Estados_arduino."3", "VISA resource name"=w517) -> ("error out"=w533:errorcluster, "VISA resource name out"=w534:refnum<visa-resource-name>)  [unwired: 6 in, 1 out]
            n203 = case shown="No Error" w533 {
              selector: w533 -> [w543 w554]
              tunnel: [w546 w554] -> w539
              tunnel: [w545 w555] -> w538
              tunnel: w534 -> [w544 w555]
              frame No Error {
                n204 = while {
                  tunnel: [w553] -> w546
                  tunnel: w544 -> [w550]
                  tunnel: [w548] -> w545
                  tunnel: w543 -> [w549]
                  stop <- w551 stop-if-true
                  n205 = property class="Instr"(reference=w550, error in=w549) -> (reference out=w548:refnum<visa-resource-name>, error out=w553:errorcluster, "Serial Settings:Number of Bytes at Serial Port"=w547:u32)
                  n206 = Equal?(x=w547, y=u32 2) -> (x = y?=w551:bool)
                }
              }
              frame Error {
              }
            }
            n207 = Unbundle By Name(w531) -> ("Retroc"=w528:refnum<vi>, "Izq"=w527:refnum<vi>, "Der"=w526:refnum<vi>, "Subir Z"=w525:refnum<vi>, "Avanzar"=w524:refnum<vi>, "Bajar Z"=w523:refnum<vi>, "Distancia"=w522:refnum<vi>, "Stop Program"=w521:refnum<vi>, "Movimiento ejecutado?"=w519:refnum<vi>)
            n208 = call "Ack_comando_arduino.vi"("error in (no error)"=w539, 10:Comandos."FH", "VISA resource name"=w538) -> ("error IO"=w530:errorcluster, "VISA resource name 2"=w537:refnum<visa-resource-name>)  [unwired: 6 in, 1 out]
            n209 = Build Array(w528, w527, w526, w525, w524, w523, w522, w521, w519) -> (w520:refnum<vi>[])
            n210 = call "Actualizar_Interfaz.vi"("error in (no error)"=w530, "Enum"=Acciones_UI."Activar", "Controls"=w520) -> ("error out"=w518:errorcluster)  [unwired: 7 in, 1 out]
            n211 = property on="Distancia Z" class="Ring (strict)"(error in=w518, "DisabledEnum"=w514) -> ()  [unwired: 1 in, 2 out]
            n212 = property on="Set coord. entrada" class="Bool"("DisabledEnum"=w514) -> ()  [unwired: 2 in, 2 out]
            n213 = property on="Set coord. OK" class="Bool"("DisabledEnum"=w514) -> ()  [unwired: 2 in, 2 out]
            n214 = property on="Set coord. NOK" class="Bool"("DisabledEnum"=w514) -> ()  [unwired: 2 in, 2 out]
            n215 = property on="Set coord. socket" class="Bool"("DisabledEnum"=w514) -> (error out=w513:errorcluster)  [unwired: 2 in, 1 out]
            n216 = Select(t=ESTADOS."Salir" ("Enum"), s=w513, f=ESTADOS."Check Button") -> (s? t:f=w536:T4)
          }
          frame "Init Refs" {
            w558 = T9."Disabled and Grayed Out" ("Disabled")
            n217 = control-ref of="Distancia"() -> (w557:refnum<vi>)
            n218 = control-ref of="Izquierda"() -> (w583:refnum<vi>)
            n219 = control-ref of="HOME"() -> (w584:refnum<vi>)
            n220 = control-ref of="Derecha"() -> (w582:refnum<vi>)
            n221 = control-ref of="STOP PROGRAM"() -> (w581:refnum<vi>)
            n222 = control-ref of="Avance"() -> (w580:refnum<vi>)
            n223 = control-ref of="COMENZAR MOVIMIENTO"() -> (w568:refnum<vi>)
            n224 = control-ref of="Baja Z"() -> (w579:refnum<vi>)
            n225 = control-ref of="Sube Z"() -> (w578:refnum<vi>)
            n226 = control-ref of="Retroceso"() -> (w577:refnum<vi>)
            n227 = control-ref of="Movimiento ejecutado?"() -> (w563:refnum<vi>)
            n228 = control-ref of="MENSAJES AL USUARIO"() -> (w561:refnum<vi>)
            n229 = control-ref of="TRAMA DE MOVIMIENTO ENVIADA"() -> (w565:refnum<vi>)
            n230 = property class="Str"(reference=w561, "Text.FontSize"=u32 30 ("Text.Font:Size"), "Text.FontBold"=TRUE ("Text.Font:Bold")) -> ()  [unwired: 1 in, 2 out]
            n231 = Bundle By Name(cluster=w587, "Comenzar mov"=w568, "Home"=w584, "Izq"=w583, "Der"=w582, "Stop Program"=w581, "Avanzar"=w580, "Bajar Z"=w579, "Distancia"=w557, "Subir Z"=w578, "Retroc"=w577, "MENSAJES AL USUARIO"=w561, "Trama enviada"=w565, "Movimiento ejecutado?"=w563) -> (w574:T12)
            n232 = Build Array(w584, w583, w582, w581, w580, w579, w557, w578, w577, w568, w563) -> (w576:refnum<vi>[])
            n233 = call "Actualizar_Interfaz.vi"("Enum"=Acciones_UI."Desactivar", "Controls"=w576) -> ()  [unwired: 8 in, 2 out]
            n234 = Build Array(w561) -> (w585:refnum<vi>[])
            n235 = call "Actualizar_Interfaz.vi"("Enum"=Acciones_UI."Activar", "Controls"=w585) -> ("Controls 2"=w567:refnum<vi>[])  [unwired: 8 in, 1 out]
            n236 = call "Actualizar_Interfaz.vi"("Enum"=Acciones_UI."Reiniciar default", "Controls"=w567) -> ()  [unwired: 8 in, 2 out]
            n237 = Select(t=ESTADOS."Salir" ("Enum"), s=w569, f=ESTADOS."Ping_Arduino") -> (s? t:f=w570:T4)
            n238 = property on="Distancia Z" class="Ring (strict)"("DisabledEnum"=w558) -> ()  [unwired: 2 in, 2 out]
            n239 = property on="Set coord. OK" class="Bool"("DisabledEnum"=w558) -> ()  [unwired: 2 in, 2 out]
            n240 = property on="Set coord. socket" class="Bool"("DisabledEnum"=w558) -> ()  [unwired: 2 in, 2 out]
            n241 = property on="Set coord. NOK" class="Bool"("DisabledEnum"=w558) -> ()  [unwired: 2 in, 2 out]
            n242 = property on="Set coord. entrada" class="Bool"("DisabledEnum"=w558) -> ()  [unwired: 2 in, 2 out]
          }
          frame "Cabezal Posicion Inicio" {
            n243 = disable-structure shown="Disabled" {
              disable-tunnel: w595 -> [w607 _]
              disable-tunnel: [w603 _] -> w594
              disable-tunnel: w593 -> [w601 _]
              disable-tunnel: w592 -> [w600 _]
              disable-tunnel: [w597 _] -> w591
              frame Disabled {
                # "ENVIO COMANDO PARA POSICION INICIO\nEL ROBOT SE EMPIEZA A MOVER A POSICION\nINICIO"
                # "LEO ESTADO EN ARDUINO"
                n244 = call "Ack_estado_Arduino.vi"("error in (no error)"=w607, "Enum"=Estados_arduino."4", "VISA resource name"=w601) -> ("error out"=w606:errorcluster)  [unwired: 6 in, 2 out]
                n245 = call "Enviar_comando.vi"("error in (no error)"=w606, "Enum"=Comandos."I", "VISA resource name"=w601) -> ("error out"=w598:errorcluster)  [unwired: 6 in, 2 out]
                n246 = Unbundle By Name(w600) -> ("MENSAJES AL USUARIO"=w599:refnum<vi>)
                n247 = property class="Str"(reference=w599, error in=w598, "Text.Text"="CABEZAL YENDO A POSICION DE INICIO") -> (error out=w597:errorcluster)  [unwired: 1 out]
                n248 = Select(t=ESTADOS."Salir", s=w597, f=ESTADOS."Terminaste posicion inicio?" ("Enum")) -> (s? t:f=w603:T4)
              }
              frame Enabled {
              }
            }
          }
          frame "Terminaste posicion inicio?" {
            n249 = disable-structure shown="Disabled" {
              disable-tunnel: [w636 _] -> w616
              disable-tunnel: w615 -> [w635 _]
              disable-tunnel: w614 -> [w623 _]
              disable-tunnel: w613 -> [w622 _]
              disable-tunnel: [w621 _] -> w612
              frame Disabled {
                # "LEO ESTADO EN ARDUINO"
                # "ESPERAR A QUE SE VAYA\nA POSICION INICIO Y NOS ENVIE EL COMANDO\n\"FI\""
                # "ESPERO COMANDO POSICION INICIO\nFINALIZADA"
                n250 = call "Ack_estado_Arduino.vi"("error in (no error)"=w623, "Enum"=Estados_arduino."5", "VISA resource name"=w622) -> ("error out"=w637:errorcluster)  [unwired: 6 in, 2 out]
                n251 = case shown="No Error" w637 {
                  selector: w637 -> [w643 w652]
                  tunnel: [w645 w652] -> w639
                  tunnel: w622 -> [w644 _]
                  frame No Error {
                    n252 = while {
                      tunnel: [w651] -> w645
                      tunnel: w644 -> [w647]
                      tunnel: w643 -> [w646]
                      stop <- w648 stop-if-true
                      # "POLLING"
                      n253 = property class="Instr"(reference=w647, error in=w646) -> (error out=w651:errorcluster, "Serial Settings:Number of Bytes at Serial Port"=w650:u32)  [unwired: 1 out]
                      n254 = Equal?(x=w650, y=u32 2) -> (x = y?=w648:bool)
                    }
                  }
                  frame Error {
                  }
                }
                n255 = call "Ack_comando_arduino.vi"("error in (no error)"=w639, 10:Comandos."FI", "VISA resource name"=w622) -> ("error IO"=w620:errorcluster)  [unwired: 6 in, 2 out]
                n256 = Unbundle By Name(w635) -> ("Retroc"=w634:refnum<vi>, "Home"=w633:refnum<vi>, "Izq"=w632:refnum<vi>, "Der"=w631:refnum<vi>, "Stop Program"=w630:refnum<vi>, "Avanzar"=w629:refnum<vi>, "Bajar Z"=w628:refnum<vi>, "Distancia"=w627:refnum<vi>, "Subir Z"=w626:refnum<vi>, "MENSAJES AL USUARIO"=w619:refnum<vi>)
                n257 = property class="Str"(reference=w619, error in=w620, "Text.Text"="CABEZAL EN POSICION DE INICIO") -> (error out=w617:errorcluster)  [unwired: 1 out]
                n258 = Build Array(w634, w633, w632, w631, w630, w629, w628, w627, w626) -> (w625:refnum<vi>[])
                n259 = call "Actualizar_Interfaz.vi"("error in (no error)"=w617, "Enum"=Acciones_UI."Activar", "Controls"=w625) -> ("error out"=w621:errorcluster)  [unwired: 7 in, 1 out]
                n260 = Select(t=ESTADOS."Salir" ("Enum"), s=w621, f=ESTADOS."Check Button") -> (s? t:f=w636:T4)
              }
              frame Enabled {
              }
            }
          }
          frame "Ping_Arduino" {
            n261 = VISA Write(VISA resource name=w658, write buffer="Q?", error in (no error)=w667) -> (return count=w670:u32, error out=w669:errorcluster)  [unwired: 1 out]
            n262 = VISA Read(VISA resource name=w658, byte count=w670, error in (no error)=w669) -> (read buffer=w665:string, error out=w664:errorcluster)  [unwired: 2 out]
            n263 = Equal?(x=w665, y="R!") -> (x = y?=w666:bool)
            n264 = case shown="True" w666 {
              tunnel: w665 -> [w683 _]
              tunnel: w664 -> [w681 w698]
              tunnel: [w680 w698] -> w656
              tunnel: w660 -> [w678 w696]
              frame False {
                n265 = Unbundle By Name(w678) -> ("MENSAJES AL USUARIO"=w677:refnum<vi>)
                n266 = xnode "Error Ring"("parameter 0"=w683) -> ("error out"=w682:errorcluster)
                n267 = property class="Str"(reference=w677, "Text.Text"="LA COMUNICACION CON ARDUINO HA FALLADO") -> ()  [unwired: 1 in, 2 out]
                n268 = Merge Errors(w682, w681) -> (w680:errorcluster)
              }
              frame True {
                n269 = Unbundle By Name(w696) -> ("Comenzar mov"=w694:refnum<vi>, "MENSAJES AL USUARIO"=w695:refnum<vi>, "Stop Program"=w691:refnum<vi>)
                n270 = Build Array(w694, w691) -> (w693:refnum<vi>[])
                n271 = call "Actualizar_Interfaz.vi"("Enum"=Acciones_UI."Activar", "Controls"=w693) -> ()  [unwired: 8 in, 2 out]
                n272 = property class="Str"(reference=w695, "Text.Text"="COMUNICACION ESTABLECIDA") -> ()  [unwired: 1 in, 2 out]
              }
            }
            n273 = case shown="\"CONFIG ESTACION\"" w653 {
              tunnel: w656 -> [w672 w673 w676]
              tunnel: [w672 w673 w675] -> w655
              tunnel: [_ _ w674] -> w654
              frame "NINGUNA", Default {
              }
              frame "MOVIMIENTO MANUAL" {
              }
              frame "CONFIG ESTACION" {
                n274 = call "Encender_led_cam.vi"("error in (no error)"=w676) -> ("error out"=w675:errorcluster, "reference out"=w674:refnum<k7>)  [unwired: 9 in]
              }
            }
            n275 = Select(t=ESTADOS."Salir" ("Enum"), s=w655, f=ESTADOS."Check Button") -> (s? t:f=w661:T4)
          }
          frame "Salir Arduino" {
            w712 = "E" ("write buffer")
            n276 = VISA Clear(VISA resource name=w707, error in (no error)=w706) -> (error out=w705:errorcluster)  [unwired: 1 out]
            n277 = VISA Write(VISA resource name=w707, write buffer=w712, error in (no error)=w705) -> (VISA resource name out=w715:refnum<visa-resource-name>, return count=w714:u32, error out=w708:errorcluster)
            n278 = VISA Read(VISA resource name=w715, byte count=w714, error in (no error)=w708) -> (read buffer=w713:string, error out=w709:errorcluster)  [unwired: 2 out]
            n279 = Equal?(x=w713, y=w712) -> (x = y?=w711:bool)
            n280 = case shown="True" w711 {
              frame False {
                n281 = xnode "Error Ring"() -> ()  [unwired: 1 out]
              }
              frame True {
                n282 = property on="MENSAJES AL USUARIO" class="Str"("Value"="VI DETENIDO CORRECTAMENTE...SALIENDO" ("MENSAJES AL USUARIO")) -> ()  [unwired: 2 in, 2 out]
                n283 = call "Time Delay"() -> ()  [unwired: 11 in, 1 out]
              }
            }
            n284 = case shown="\"CONFIG ESTACION\"" w699 {
              tunnel: w703 -> [_ _ w722]
              tunnel: [_ _ w721] -> w701
              tunnel: [_ _ w720] -> w702
              frame "NINGUNA", Default {
              }
              frame "MOVIMIENTO MANUAL" {
              }
              frame "CONFIG ESTACION" {
                n285 = call "Apagar_led_cam.vi"("DNVideoX"=w722) -> ("error out"=w721:errorcluster, "reference out"=w720:refnum<k7>)  [unwired: 9 in]
              }
            }
            n286 = Close Reference(reference=w702, error in (no error)=w701) -> (error out=w700:errorcluster)
            n287 = Merge Errors(w700, w709) -> (w710:errorcluster)
          }
        }
        "ESTADO FSM" <- w33
        "MOVIMIENTO SOLICITADO" <- w37
        n288 = Equal?(x=w33, y=ESTADOS."Salir") -> (x = y?=w30:bool)
        n289 = Or(x=w31, y=w30) -> (x .or. y?=w34:bool)
      }
    }
    frame Error {
    }
  }
  "error out" <- w4
  "Coordenadas_estacion_outpu" <- w2
